vi "AR-Axis-get-positions.vi"(7 "Select":enum16{"X Axis", "Y Axis", "Both"}(ring), 8 "error in":errorcluster, 10 "Axis params":T1={"X"={"Device (dev axis)"="1 3", "Lockstep Group (1)"=1, "Units"=enum."millimeters", "Microstep Size"=4.21875, "Move (units)"=0.0, "Direction(-1,1)"=1, "Speed (units/s)"=1500.0}, "Y"={"Device (dev axis)"="1", "Lockstep Group (1)"=1, "Units"=enum."millimeters", "Microstep Size"=0.496094, "Move (units)"=0.0, "Direction(-1,1)"=1, "Speed (units/s)"=45.0}}, 11 "Port In":refnum<visa-resource-name>) -> (0 "error out":errorcluster, 1 "Y Pos":dbl, 2 "X Pos":dbl, 3 "Port Out":refnum<visa-resource-name>)   [LabVIEW 2021]
uses:
  Controls/AR-axis-parameters.ctl
  Automation/Zaber Stage/Controls/Zaber-parameters.ctl
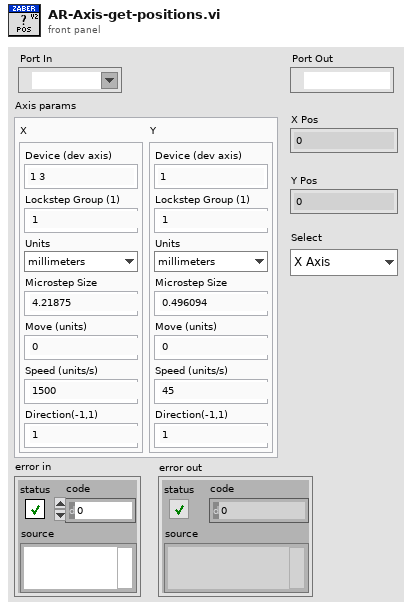
[diagram p1: front panel]
types:
  T1 = typedef "AR-axis-parameters.ctl" = cluster{"X":T2, "Y":T2}
  T2 = typedef "Zaber-parameters.ctl" = cluster{"Device (dev axis)":string, "Lockstep Group (1)":u8, "Units":enum16{"microsteps", "microns", "millimeters", "inches", "degrees"}, "Microstep Size":dbl, "Move (units)":dbl, "Direction(-1,1)":i32, "Speed (units/s)":dbl}
  T3 = enum16{"microsteps", "microns", "millimeters", "inches", "degrees"}
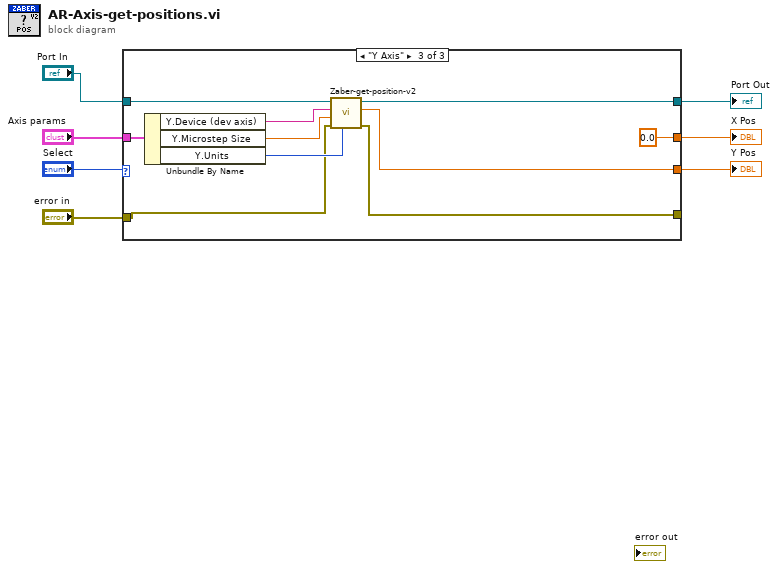
[diagram p0: block diagram]
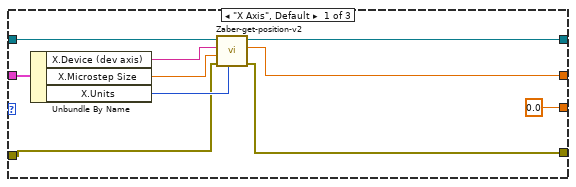
[diagram p2: hidden frame]
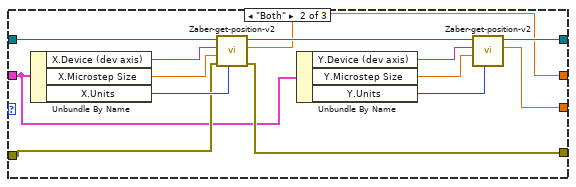
[diagram p3: hidden frame]
diagram:
  n1 = case shown="\"Y Axis\"" "Select" {
    tunnel: "Port In" -> [w17 w31 w41]
    tunnel: "Axis params" -> [w16 w25 w40]
    tunnel: "error in" -> [w12 w27 w36]
    tunnel: [w11 w26 w35] -> _
    tunnel: [w10 w20 w34] -> w3
    tunnel: [0.0 ("Position") w19 w33] -> w2
    tunnel: [w9 w18 0.0 ("Position")] -> w1
    frame "X Axis", Default {
      n2 = Unbundle By Name(w16) -> ("X.Device (dev axis)"=w15:string, "X.Microstep Size"=w14:dbl, "X.Units"=w13:T3)
      n3 = call "Zaber-get-position-v2.vi"("Units"=w13, "error in"=w12, "Microstep Size"=w14, "Device and Axis"=w15, "Port In"=w17) -> ("error out"=w11:errorcluster, "Position"=w9:dbl, "Port Out"=w10:refnum<visa-resource-name>)  [unwired: 4 in]
    }
    frame "Both" {
      n4 = Unbundle By Name(w25) -> ("X.Device (dev axis)"=w30:string, "X.Microstep Size"=w29:dbl, "X.Units"=w28:T3)
      n5 = call "Zaber-get-position-v2.vi"("Units"=w28, "error in"=w27, "Microstep Size"=w29, "Device and Axis"=w30, "Port In"=w31) -> ("error out"=w26:errorcluster, "Position"=w18:dbl, "Port Out"=w21:refnum<visa-resource-name>)  [unwired: 4 in]
      n6 = Unbundle By Name(w25) -> ("Y.Device (dev axis)"=w22:string, "Y.Microstep Size"=w23:dbl, "Y.Units"=w24:T3)
      n7 = call "Zaber-get-position-v2.vi"("Units"=w24, "Microstep Size"=w23, "Device and Axis"=w22, "Port In"=w21) -> ("Position"=w19:dbl, "Port Out"=w20:refnum<visa-resource-name>)  [unwired: 5 in, 1 out]
    }
    frame "Y Axis" {
      n8 = Unbundle By Name(w40) -> ("Y.Device (dev axis)"=w39:string, "Y.Microstep Size"=w38:dbl, "Y.Units"=w37:T3)
      n9 = call "Zaber-get-position-v2.vi"("Units"=w37, "error in"=w36, "Microstep Size"=w38, "Device and Axis"=w39, "Port In"=w41) -> ("error out"=w35:errorcluster, "Position"=w33:dbl, "Port Out"=w34:refnum<visa-resource-name>)  [unwired: 4 in]
    }
  }
  "Port Out" <- w3
  "X Pos" <- w1
  "Y Pos" <- w2
